vi "ReadCmd.vi"(7 "Read Count":u32, 8 "error in (no error)":errorcluster, 9 "Cmd":u8, 10 "Address":u8, 11 "VISA Refnum in":refnum<visa-resource-name>) -> (0 "error out":errorcluster, 2 "Output":string, 3 "VISA Refnum out":refnum<visa-resource-name>, 5 "Valid":bool)   [LabVIEW 2015, in "Ion Motion Roboclaw.lvlib"]
uses:
  <instrlib>/Ion Motion Roboclaw/Ion Motion Roboclaw.lvlib
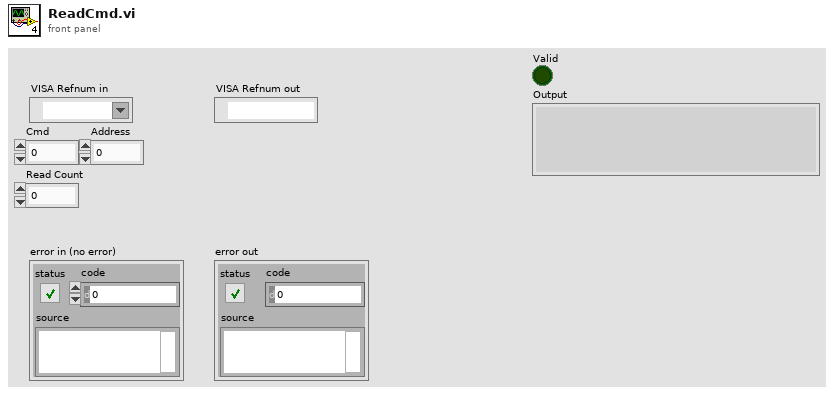
[diagram p1: front panel]
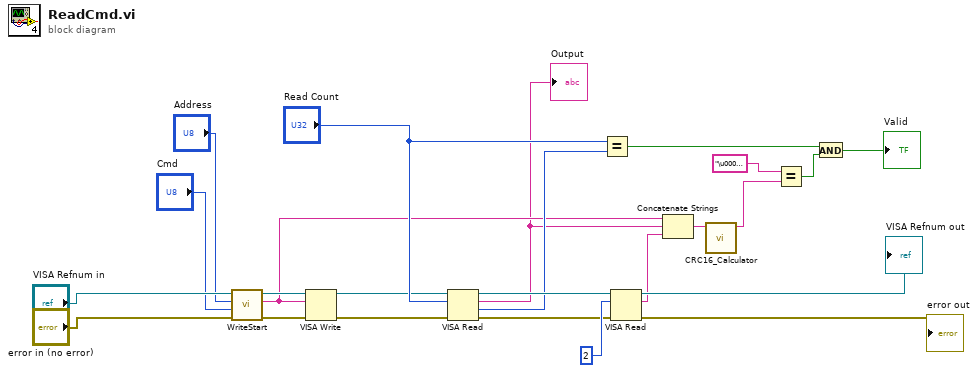
[diagram p0: block diagram]
diagram:
  n1 = call <instrlib>:"WriteStart.vi"("error in (no error)"="error in (no error)", "Cmd"="Cmd", "Address"="Address", "VISA Refnum in"="VISA Refnum in") -> ("error out"=w5:errorcluster, "String Out"=w3:string, "VISA Refnum out"=w4:refnum<visa-resource-name>)  [unwired: 5 in]
  n2 = VISA Write(VISA resource name=w4, write buffer=w3, error in (no error)=w5) -> (VISA resource name out=w7:refnum<visa-resource-name>, error out=w6:errorcluster)  [unwired: 1 out]
  n3 = VISA Read(VISA resource name=w7, byte count="Read Count", error in (no error)=w6) -> (VISA resource name out=w20:refnum<visa-resource-name>, read buffer=w2:string, return count=w18:u32, error out=w19:errorcluster)
  "Output" <- w2
  n4 = Equal?(x="Read Count", y=w18) -> (x = y?=w17:bool)
  n5 = VISA Read(VISA resource name=w20, byte count=u32 2, error in (no error)=w19) -> (VISA resource name out=→"VISA Refnum out":refnum<visa-resource-name>, read buffer=w21:string, error out=→"error out":errorcluster)  [unwired: 1 out]
  n6 = Concatenate Strings(w3, w2, w21) -> (w1:string)
  n7 = call <instrlib>:"CRC16_Calculator.vi"("String in"=w1) -> ("CRC16 out"=w10:string)  [unwired: 8 in, 2 out]
  n8 = Equal?(x="\u0000\u0000", y=w10) -> (x = y?=w16:bool)
  n9 = And(x=w17, y=w16) -> (x .and. y?=→"Valid":bool)
